vi "get channel strings.vi"(11 "line item in":T2) -> (3 "Tag Names":T1)   [LabVIEW 2014, in "Tagbus PID Module editor node.lvclass"]
uses:
  Tagbus PID Module editor node.lvclass
  PID array element.ctl
  module/configuration/PID Loop/String Parameters.ctl
  module/configuration/PID Loop.lvclass
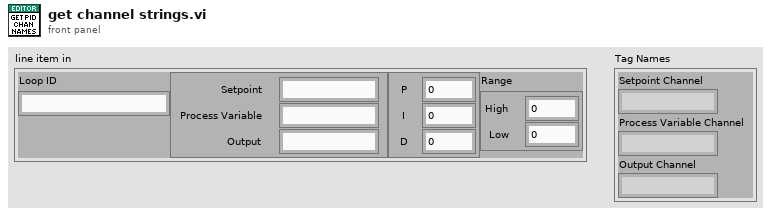
[diagram p1: front panel]
types:
  T1 = cluster{"Setpoint Channel":string, "Process Variable Channel":string, "Output Channel":string}
  T2 = typedef "Tagbus PID Module editor node.lvclass/PID array element.ctl" = cluster{"Loop ID":string, "Tags":cluster{"Setpoint":string, "Process Variable":string, "Output":string}, "Gains":cluster{"P":dbl, "I":dbl, "D":dbl}, "Range":cluster{"High":dbl, "Low":dbl}}
  T3 = typedef "PID Loop.lvclass/String Parameters.ctl" = enum16{"Setpoint", "Process Variable", "Output", "Proportional Gain", "Integral Time", "Derivative Time", "Range High", "Range Low"}
  T4 = cluster{"Parameter String":string, "Parameter String":string, "Parameter String":string}
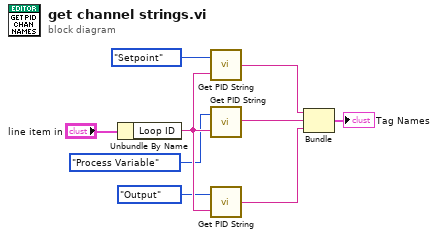
[diagram p0: block diagram]
diagram:
  n1 = Unbundle By Name("line item in") -> ("Loop ID"=w7:string)
  n2 = call "Get PID String.vi"("PID Loop ID"=w7, "PID Parameter"=String_Parameters."Setpoint") -> ("Parameter String"=w4:string)
  n3 = call "Get PID String.vi"("PID Loop ID"=w7, "PID Parameter"=String_Parameters."Process Variable") -> ("Parameter String"=w3:string)
  n4 = call "Get PID String.vi"("PID Loop ID"=w7, "PID Parameter"=String_Parameters."Output") -> ("Parameter String"=w2:string)
  n5 = Bundle("Parameter String"=w4, "Parameter String"=w3, "Parameter String"=w2) -> (→"Tag Names":T4)  [unwired: 1 in]
